vi "LVDimInterface.test simple client.vi"() -> ()   [LabVIEW 2015, in "LVDimInterface.lvlib"]
doc: "This is an example of a DIM client receiving service data via a message queue."
uses:
  LVDimInterface.lvlib
  LVDimInterface.dim service type.ctl
  LVDimInterface.dic_info_service_queue.vi
panel:
  out "error out":errorcluster
  out "callBackID":i32
  out "no link":bool
  out "serviceData":i32
  out "serviceSize":i32
  in  "serviceName":string="testBuffer"
  out "receivedCounter":i32
  in  "stop":bool
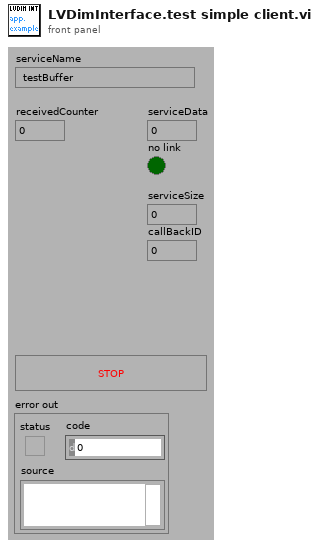
[diagram p1: front panel]
types:
  T1 = typedef "LVDimInterface.lvlib/LVDimInterface.dim service type.ctl" = u16
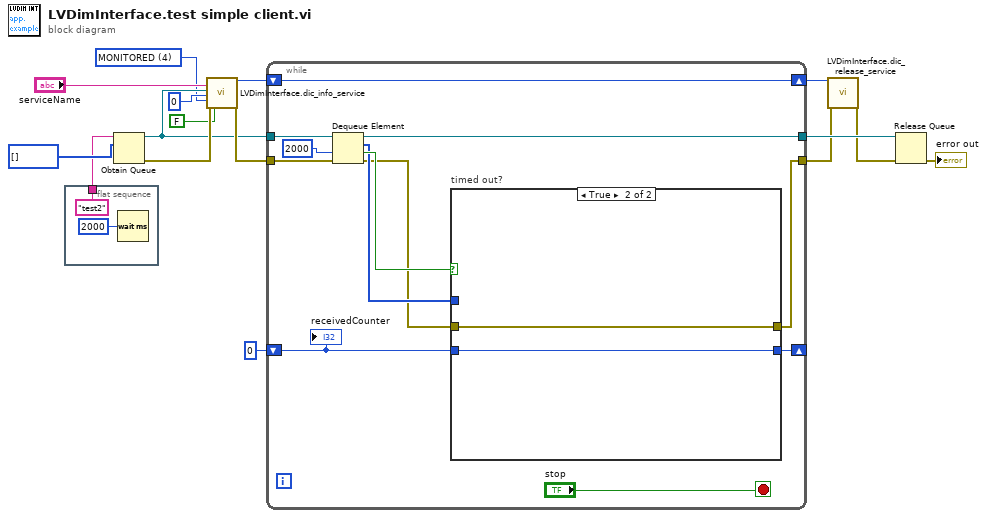
[diagram p0: block diagram]
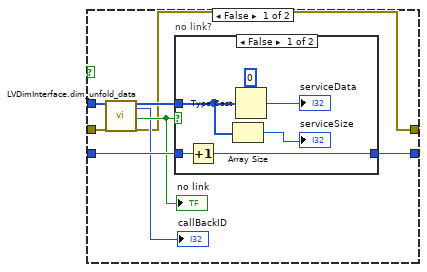
[diagram p2: hidden frame]
diagram:
  w4 = T1 4 items=["ONCE_ONLY"=1, "TIMED"=2, "MONITORED"=4] ("serviceType")
  n1 = flat-sequence {
    tunnel: ["test2" ("name (unnamed)")] -> w2
    frame #0 {
      n2 = Wait (ms)(milliseconds to wait=u32 2000) -> ()  [unwired: 1 out]
    }
  }
  n3 = Obtain Queue(name (unnamed)=w2, element data type=i8[] []) -> (queue out=w6:refnum<queue>, error out=w13:errorcluster)  [unwired: 3 in, 1 out]
  n4 = call-poly "LVDimInterface.dic_info_service.vi"("serviceName"="serviceName", "queueRef"=w6, "timeout [s]"=0, "serviceType"=w4, "error in (no error)"=w13, "stamped"=FALSE) -> ("callBackID"=w16:i32, "error out"=w12:errorcluster)  [unwired: 12 in]
  n5 = while {
    tunnel: w6 -> [w30]
    tunnel: [w28] -> w15
    shift-right: [w24] -> _
    shift-left: 0 -> [w25]
    tunnel: w12 -> [w23]
    tunnel: [w19] -> w10
    shift-right: [w21] -> w11
    shift-left: w16 -> [w21]
    stop <- "stop" stop-if-true
    n6 = Dequeue Element(queue=w30, timeout in ms (-1)=2000, error in (no error)=w23) -> (queue out=w28:refnum<queue>, element=w22:i8[], timed out?=w27:bool, error out=w20:errorcluster)
    n7 = case "timed out?" shown="True" w27 {
      tunnel: [w37 w47] -> w24
      tunnel: w25 -> [w38 w47]
      tunnel: w22 -> [w35 _]
      tunnel: w20 -> [w32 w46]
      tunnel: [w31 w46] -> w19
      frame False {
        n8 = call "LVDimInterface.dim_unfold_data.vi"("rawData"=w35, "error in (no error)"=w32) -> ("data"=w36:i8[], "callBackID"=→"callBackID":i32, "no link"=w34:bool, "error out"=w31:errorcluster)  [unwired: 14 in]
        "no link" <- w34
        n9 = case "no link?" shown="False" w34 {
          tunnel: w38 -> [w44 w45]
          tunnel: [w43 w45] -> w37
          tunnel: w36 -> [w40 _]
          frame False {
            n10 = Increment(x=w44) -> (x+1=w43:i32)
            n11 = Array Size(array=w40) -> (size(s)=→"serviceSize":i32)
            n12 = Type Cast(type=0, x=w40) -> (*(type *) &x=→"serviceData":i32)
          }
          frame True {
          }
        }
      }
      frame True {
      }
    }
    "receivedCounter" <- w25
  }
  n13 = call "LVDimInterface.dic_release_service.vi"("callBackID"=w11, "error in (no error)"=w10) -> ("error out"=w9:errorcluster)  [unwired: 17 in]
  n14 = Release Queue(queue=w15, error in (no error)=w9) -> (error out=→"error out":errorcluster)  [unwired: 1 in, 2 out]
